vi "Read.vi"(6 "prioritize Cache? (F)":bool, 7 "Qualified Name":string, 8 "error in (no error)":errorcluster, 9 "Default Values":variant[](array[variant]), 10 "keys in":string[](array[string]), 11 "ConfigManager in":refnum<class "ConfigManager.lvclass">) -> (0 "error out":errorcluster, 1 "Values":variant[](array[variant]), 2 "keys":string[](array[string]), 3 "ConfigManager out":refnum<class "ConfigManager.lvclass">)   [LabVIEW 2013, in "SMOConfig.lvlib" / "ConfigManager.lvclass"]
uses:
  ConfigManager.lvclass
  ConfigManager.lvclass/ConfigManager.ctl
  Encoding/Encoding.lvclass
  Encryption/Encryption.lvclass
  Serializer/Serializer.lvclass
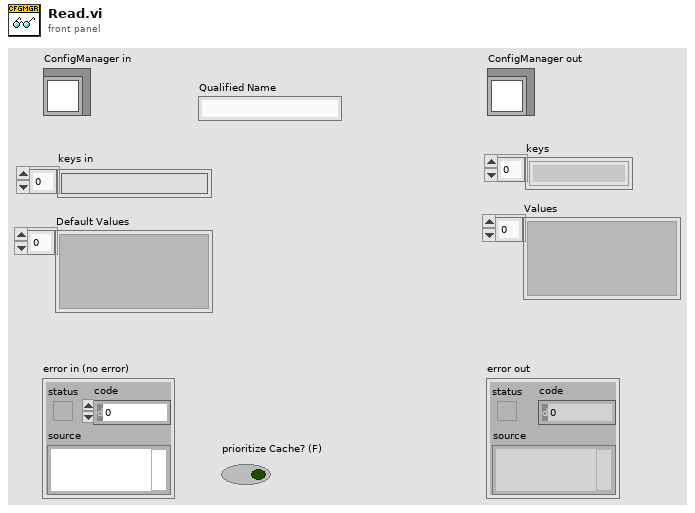
[diagram p1: front panel]
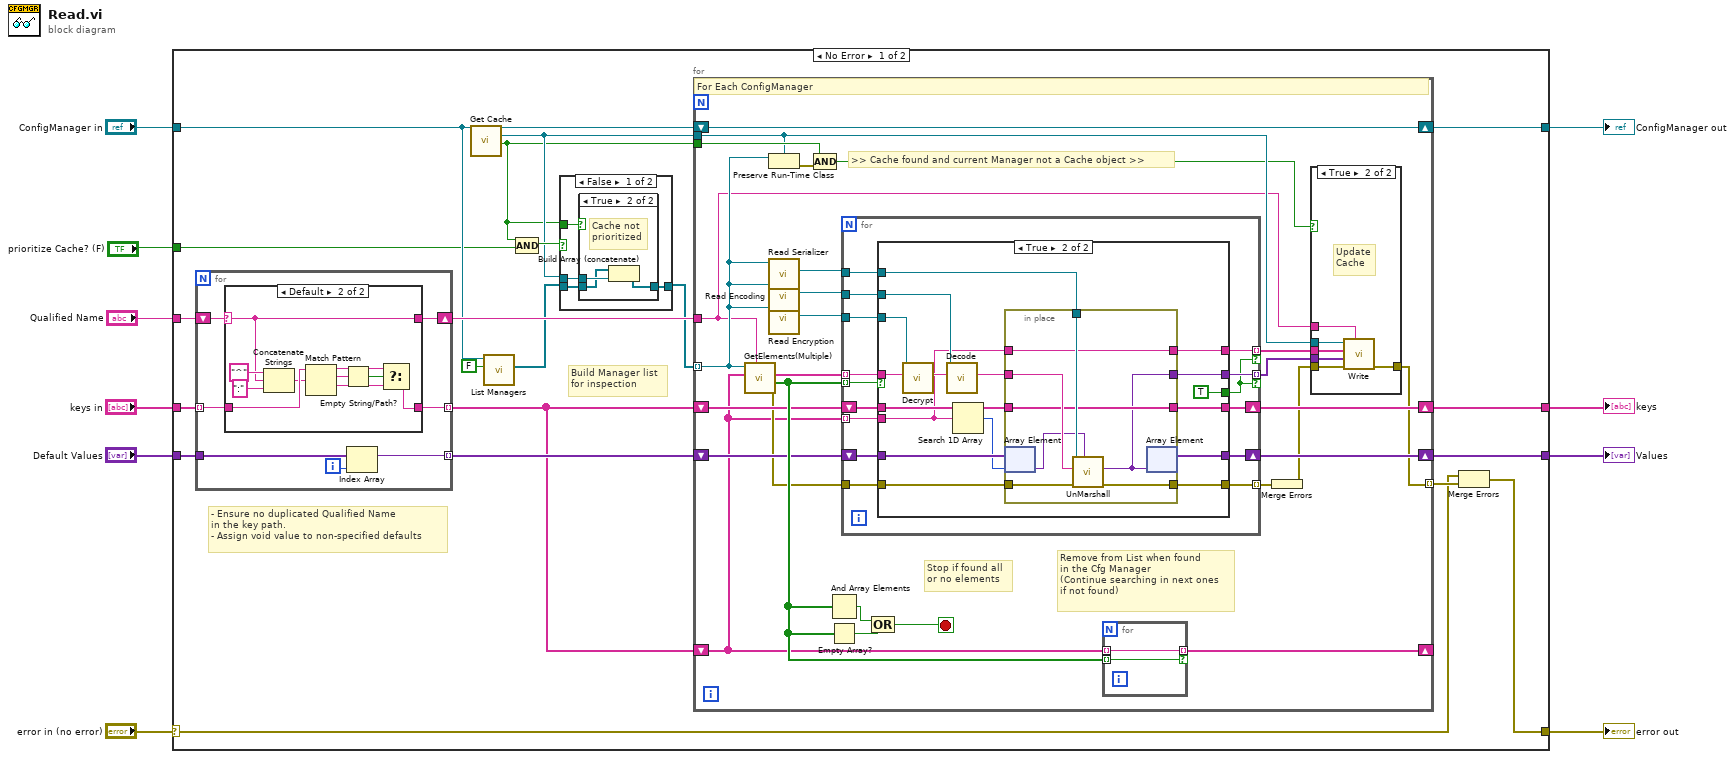
[diagram p0: block diagram]
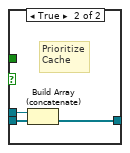
[diagram p3: hidden frame]
diagram:
  n1 = case shown="No Error" "error in (no error)" {
    selector: "error in (no error)" -> [w26 w144]
    tunnel: [w25 w144] -> w9
    tunnel: [w13 w143] -> w7
    tunnel: "ConfigManager in" -> [w19 w143]
    tunnel: "keys in" -> [w24 w141]
    tunnel: "Default Values" -> [w30 w142]
    tunnel: [w29 w142] -> w4
    tunnel: [w28 w141] -> w3
    tunnel: "Qualified Name" -> [w22 _]
    tunnel: "prioritize Cache? (F)" -> [w15 _]
    frame No Error {
      # "Build Manager list\nfor inspection"
      # "- Ensure no duplicated Qualified Name\nin the key path.\n- Assign void value to non-specified defaults"
      n2 = for {
        tunnel: w30 -> [w48]
        tunnel: [w47] -> w31 mode=indexing
        tunnel: w24 -> [w46] mode=indexing
        tunnel: [w43] -> w23 mode=indexing
        shift-right: [w44] -> w21
        shift-left: w22 -> [w45]
        i -> [w49]
        n3 = case shown="Default" w45 {
          selector: w45 -> [w51 w58]
          tunnel: w46 -> [w50 w61]
          tunnel: [w51 w58] -> w44
          tunnel: [w50 w52] -> w43
          frame "" {
          }
          frame Default {
            n4 = Concatenate Strings("^" ("string"), w58, ":" ("string")) -> (w60:string)
            n5 = Match Pattern(string=w61, regular expression=w60) -> (before substring=w55:string, match substring=w57:string, after substring=w54:string)  [unwired: 1 in, 1 out]
            n6 = Empty String/Path?(string/path=w57) -> (empty?=w56:bool)
            n7 = Select(t=w55, s=w56, f=w54) -> (s? t:f=w52:string)
          }
        }
        n8 = Index Array(array=w48, index=w49) -> (element=w47:variant)
      }
      n9 = call-dynamic "Get Cache.vi"("ConfigManager in"=w19) -> ("found?"=w11:bool, "Cache"=w12:refnum<class "ConfigManager.Cache.lvclass">, "ConfigManager out"=w14:refnum<class "ConfigManager.lvclass">)  [unwired: 8 in]
      n10 = call-dynamic "List Managers.vi"("Include Cache? (F)"=FALSE, "SMOConfigManager in"=w19) -> ("List"=w18:refnum<class "ConfigManager.lvclass">[])  [unwired: 8 in, 1 out]
      n11 = Compound Arithmetic op=AND(w11, w15) -> (w16:bool)
      n12 = case shown="False" w16 {
        tunnel: w12 -> [w34 w42]
        tunnel: w18 -> [w33 w41]
        tunnel: [w32 w40] -> w17
        tunnel: w11 -> [w35 _]
        frame False {
          n13 = case shown="True" w35 {
            tunnel: w34 -> [_ w39]
            tunnel: w33 -> [w36 w38]
            tunnel: [w36 w37] -> w32
            frame False {
              # "No cache\nfound"
            }
            frame True {
              # "Cache not\nprioritized"
              n14 = Build Array (concatenate)(w38, w39) -> (w37:refnum<class "ConfigManager.lvclass">[])
            }
          }
        }
        frame True {
          # "Prioritize\nCache"
          n15 = Build Array (concatenate)(w42, w41) -> (w40:refnum<class "ConfigManager.lvclass">[])
        }
      }
      n16 = for {
        tunnel: w17 -> [w71] mode=indexing
        shift-right: [w83] -> _
        shift-left: w23 -> [w74]
        shift-right: [w79] -> w29
        shift-left: w31 -> [w82]
        shift-right: [w80] -> w28
        shift-left: w23 -> [w81]
        tunnel: [w65] -> w27 mode=indexing
        tunnel: w21 -> [w63]
        shift-right: [w72] -> w13
        shift-left: w14 -> [w72]
        tunnel: w12 -> [w68]
        tunnel: w11 -> [w69]
        stop <- w85 stop-if-true
        # ">> Cache found and current Manager not a Cache object >>"
        # "Remove from List when found\nin the Cfg Manager\n(Continue searching in next ones\nif not found)"
        # "Stop if found all\nor no elements"
        # "For Each ConfigManager"
        n17 = call-dynamic "GetElements(Multiple).vi"("Qualified Name"=w63, "keys"=w74, "SMOConfigManager in"=w71) -> ("error out"=w76:errorcluster, "Found"=w84:bool[], "Values"=w88:string[])  [unwired: 5 in, 1 out]
        n18 = Preserve Run-Time Class(object in=w71, 2:w68) -> (error out=w70:errorcluster)  [unwired: 1 in, 1 out]
        n19 = call "Read Serializer.vi"("ConfigManager in"=w71) -> ("Serializer"=w77:refnum<class "Serializer.lvclass">)  [unwired: 9 in, 1 out]
        n20 = call "Read Encoding.vi"("ConfigManager in"=w71) -> ("Encoding"=w78:refnum<class "Encoding.lvclass">)  [unwired: 9 in, 1 out]
        n21 = call "Read Encryption.vi"("ConfigManager in"=w71) -> ("Encryption"=w73:refnum<class "Encryption.lvclass">)  [unwired: 9 in, 1 out]
        n22 = Compound Arithmetic op=AND(w69, w70) -> (w62:bool)
        n23 = And Array Elements(Boolean array=w84) -> (logical AND=w86:bool)
        n24 = Empty Array?(array=w84) -> (empty?=w87:bool)
        n25 = for {
          tunnel: w88 -> [w112] mode=indexing
          tunnel: w77 -> [w111]
          tunnel: w78 -> [w110]
          tunnel: w84 -> [w109] mode=indexing
          shift-right: [w106] -> w80
          shift-left: w81 -> [w108]
          shift-right: [w105] -> w79
          shift-left: w82 -> [w107]
          tunnel: w76 -> [w104]
          tunnel: [w103] -> w75 mode=indexing
          tunnel: w74 -> [w102] mode=indexing
          tunnel: w73 -> [w101]
          tunnel: [w100] -> w66 mode=indexing if=w98
          tunnel: [w99] -> w67 mode=indexing if=w98
          n26 = case shown="True" w109 {
            tunnel: w112 -> [_ w122]
            tunnel: w111 -> [_ w128]
            tunnel: w110 -> [_ w132]
            tunnel: w108 -> [w115 w125]
            tunnel: w107 -> [w114 w131]
            tunnel: [w115 w126] -> w106
            tunnel: [w114 w130] -> w105
            tunnel: w104 -> [w113 w124]
            tunnel: [w113 w123] -> w103
            tunnel: w102 -> [_ w117]
            tunnel: w101 -> [_ w120]
            tunnel: [_ w119] -> w100
            tunnel: [_ w118] -> w99
            tunnel: [_ TRUE] -> w98
            frame False {
            }
            frame True {
              n27 = call-dynamic "Decrypt.vi"("Encrypted String"=w122, "Encryption in"=w120) -> ("String"=w121:string)  [unwired: 8 in, 1 out]
              n28 = call-dynamic "Decode.vi"("Encoded String"=w121, "CfgEncoding in"=w132) -> ("String"=w127:string)  [unwired: 8 in, 1 out]
              n29 = Search 1D Array(1D array=w125, element=w117) -> (index of element=w129:i32)  [unwired: 1 in]
              n30 = in-place {
                in-place-border: w128 -> [w140]
                in-place-border: w127 -> [w139]
                in-place-border: [w137] -> w126
                in-place-border: w125 -> [w137]
                in-place-border: w124 -> [w136]
                in-place-border: [w135] -> w123
                in-place-border: [w134] -> w119
                in-place-border: [w133] -> w118
                in-place-border: w117 -> [w133]
                n31 = in-place-array #1(w131, w129) -> (w138:variant)
                n32 = call-dynamic "UnMarshall.vi"("Type"=w138, "error in (no error)"=w136, "String"=w139, "Serializer in"=w140) -> ("error out"=w135:errorcluster, "Variant"=w134:variant)  [unwired: 5 in, 1 out]
                n33 = in-place-array #1(w134) -> (w130:variant[])  [unwired: 1 out]
              }
            }
          }
        }
        n34 = Compound Arithmetic op=OR(w86, w87) -> (w85:bool)
        n35 = for {
          tunnel: w74 -> [w97] mode=indexing
          tunnel: w84 -> [w96] mode=indexing
          tunnel: [w97] -> w83 mode=indexing if=w96
        }
        n36 = Merge Errors(w75) -> (w64:errorcluster)
        n37 = case shown="True" w62 {
          tunnel: w68 -> [_ w95]
          tunnel: w67 -> [_ w94]
          tunnel: w66 -> [_ w93]
          tunnel: [w89 w90] -> w65
          tunnel: w64 -> [w89 w92]
          tunnel: w63 -> [_ w91]
          frame False {
          }
          frame True {
            # "Update\nCache"
            n38 = call "Write.vi"("Qualified Name"=w91, "error in (no error)"=w92, "Values"=w93, "keys"=w94, "ConfigManager in"=w95) -> ("error out"=w90:errorcluster)  [unwired: 4 in, 2 out]
          }
        }
      }
      n39 = Merge Errors(w26, w27) -> (w25:errorcluster)
    }
    frame Error {
    }
  }
  "error out" <- w9
  "ConfigManager out" <- w7
  "Values" <- w4
  "keys" <- w3
